vi "Write 1D U16.vi"(7 "count (-1: all)":i64=-1 format="%d elements", 8 "error in (no error)":errorcluster, 9 "offset (0)":u64 format="%d bytes", 10 "buffer in":u16[](array[numeric]), 11 "Buffer in":refnum<class "Buffer.lvclass">) -> (0 "error out":errorcluster, 1 "offset out":u64 format="%d bytes", 2 "buffer out":u16[](array[numeric]), 3 "Buffer out":refnum<class "Buffer.lvclass">)   [LabVIEW 2017, in "DSF Core.lvlib" / "Buffer.lvclass"]
uses:
  Buffer.lvclass
  C:/Program Files (x86)/National Instruments/LabVIEW 2017/vi.lib/NI/Memory Manager/Classes/Pointer/Pointer.lvclass
  <vilib>/NI/Memory Manager/Classes/Pointer/Pointer.lvclass/Pointer.ctl
  <vilib>/NI/Memory Manager/Classes/Pointer/Public/Write/Write (1D U16).vi
  <vilib>/NI/Memory Manager/Classes/Pointer/Public/Write (No Check)/Write (No Check 1D U16).vi
  <vilib>/NI/Memory Manager/Classes/Pointer/Protected/Parameter Checking/Check Null Pointer.vi
  <vilib>/NI/Memory Manager/Classes/Pointer/Protected/Parameter Checking/Check Subset (Power of 2).vi
  <vilib>/NI/Memory Manager/Classes/Pointer/API/Accessors/Get Address.vi
  <vilib>/NI/Memory Manager/Classes/Pointer/Protected/Errors.vi
  <vilib>/NI/Memory Manager/Classes/Pointer/Protected/Error VIs/Null Pointer.vi
  <vilib>/NI/Memory Manager/Classes/Pointer/Protected/Error VIs/Out of Bounds.vi
  <vilib>/NI/Memory Manager/Classes/Pointer/API/Accessors/Get Size.vi
  <vilib>/NI/Memory Manager/Classes/Pointer/Private/Count to Size.vi
  <vilib>/NI/Memory Manager/Classes/Pointer/Protected/Error Building/Create Error.vi
  <vilib>/NI/Memory Manager/VIs/Write String into Source.vi
  <vilib>/NI/Memory Manager/Classes/Pointer/Protected/Error Building/Write Pointer Size.vi
  <vilib>/NI/Memory Manager/VIs/Write Number into Source.vi
  <vilib>/NI/Memory Manager/VIs/VIs for Poly/Write U64 into Source.vi
  <vilib>/NI/Memory Manager/Constants/Constants.vi
  <vilib>/NI/Memory Manager/Constants/Library Name.vi
  <vilib>/NI/Memory Manager/Classes/Pointer/Protected/Error Building/Get Error Info.vi
  <vilib>/NI/Memory Manager/VIs/Create Error Cluster.vi
  <vilib>/NI/Memory Manager/VIs/VIs for Poly/Create Error Cluster (256B).vi
  <vilib>/NI/Memory Manager/VIs/Set Error Status.vi
  <vilib>/NI/Memory Manager/VIs/Set Error Code.vi
  <vilib>/NI/Memory Manager/VIs/Set Error Source.vi
  <vilib>/NI/Memory Manager/Classes/Pointer/Pointer.lvclass
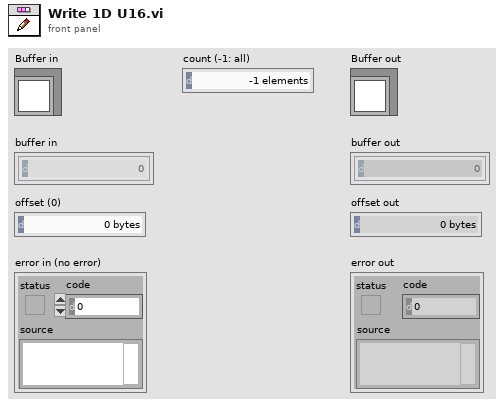
[diagram p1: front panel]
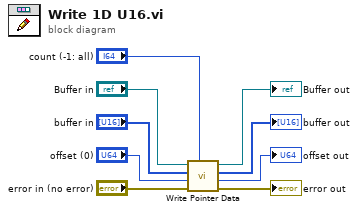
[diagram p0: block diagram]
diagram:
  n1 = call-poly <vilib>:"Write Pointer Data.vi"("count (-1: all)"="count (-1: all)", "error in (no error)"="error in (no error)", "offset (0)"="offset (0)", "buffer in"="buffer in", "Pointer in"="Buffer in") -> ("error out"=→"error out":errorcluster, "offset out"=→"offset out":u64, "buffer out"=→"buffer out":u16[], "Pointer out"=→"Buffer out":refnum<class "Buffer.lvclass">)  [unwired: 3 in]
